vi "TimeGating.vi"(2 "Counts":u32[](array[numeric]), 3 "Line Intensity in":u32[][](array[numeric]), 4 "CursorPos min out":u16, 5 "CursorPos max out":u16, 6 "Time Resolution\n(ms/pixel)":dbl, 7 "RAW data":T1) -> (0 "Counts out":u32[](array[numeric]), 1 "Line Intensity out":u32[][](array[numeric]))   [LabVIEW 2009]
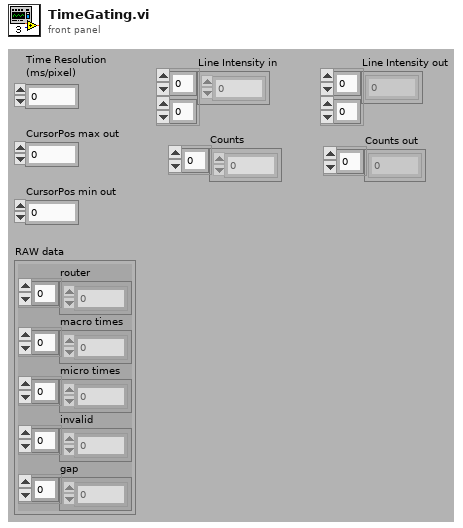
[diagram p1: front panel]
types:
  T1 = cluster{"router":u8[], "macro times":dbl[], "micro times":u16[], "invalid":dbl[], "gap":dbl[]}
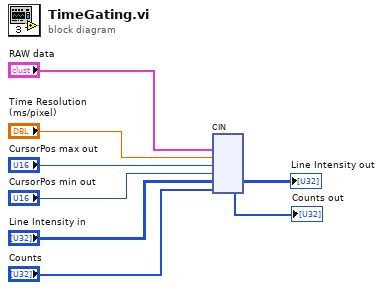
[diagram p0: block diagram]
diagram:
  n1 = cin("RAW data", "Time Resolution\n(ms/pixel)", "CursorPos max out", "CursorPos min out", "Line Intensity in", "Counts") -> (→"Line Intensity out":u32[][], →"Counts out":u32[])  [unwired: 4 in]
